vi "pb_count_boards.vi"(8 "error in (no error)":errorcluster, 11 "path in":path=path "C:/SpinCore/SpinAPI/lib32/spinapi.dll") -> (0 "error out":errorcluster, 3 "path out":path, 10 "num_boards":i32)   [LabVIEW 2016]
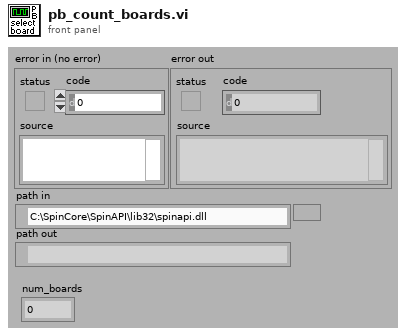
[diagram p1: front panel]
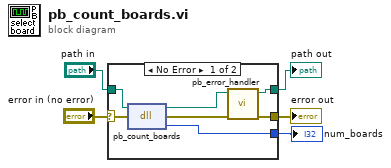
[diagram p0: block diagram]
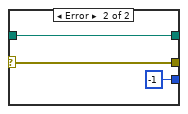
[diagram p2: hidden frame]
diagram:
  n1 = case shown="No Error" "error in (no error)" {
    selector: "error in (no error)" -> [w12 w15]
    tunnel: [w7 w15] -> w4
    tunnel: "path in" -> [w11 w14]
    tunnel: [w9 w14] -> w2
    tunnel: [w6 -1 ("board_num")] -> w1
    frame No Error {
      n2 = dll-call lib="C:/SpinCore/SpinAPI/lib32/spinapi.dll" fn="pb_count_boards" label="pb_count_board"(path in=w11, error in=w12) -> (path out=w10:path, error out=w8:errorcluster, "return type"=w6:i32)  [unwired: 1 in]
      n3 = call "pb_error_handler.vi"("error in (no error)"=w8, "path in"=w10) -> ("error out"=w7:errorcluster, "path out"=w9:path)  [unwired: 1 in, 7 out]
    }
    frame Error {
    }
  }
  "error out" <- w4
  "path out" <- w2
  "num_boards" <- w1
